vi "Write Microscope Configuration.vi"(8 "error in (no error)":errorcluster, 10 "Microscope Configuration":T1={"Serial Port"="COM2"}, 11 "TE2000 in":refnum<class "TE2000.lvclass">) -> (0 "error out":errorcluster, 3 "TE2000 out":refnum<class "TE2000.lvclass">)   [LabVIEW 2014, in "TE2000.lvlib" / "TE2000.lvclass"]
uses:
  TE2000.lvclass
  Resources/Type Defs/Microscope Configuration.ctl
  TE2000.lvclass/TE2000.ctl
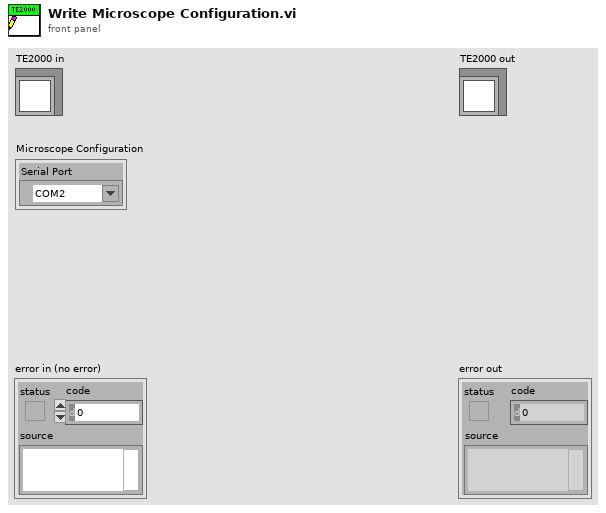
[diagram p1: front panel]
types:
  T1 = typedef "Microscope Configuration.ctl" = cluster{"Serial Port":refnum<visa-resource-name>}
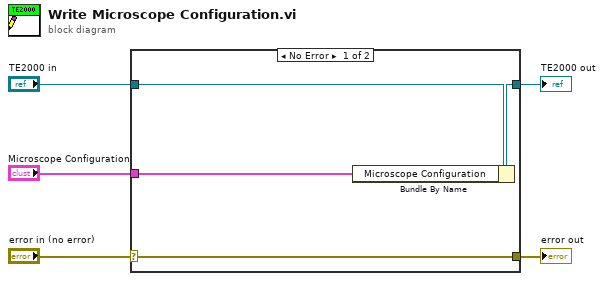
[diagram p0: block diagram]
diagram:
  n1 = case shown="No Error" "error in (no error)" {
    selector: "error in (no error)" -> [w9 w10]
    tunnel: [w9 w10] -> w4
    tunnel: [w7 w11] -> w2
    tunnel: "TE2000 in" -> [w8 w11]
    tunnel: "Microscope Configuration" -> [w6 _]
    frame No Error {
      n2 = Bundle By Name(cluster=w8, "Microscope Configuration"=w6) -> (w7:refnum<class "TE2000.lvclass">)
    }
    frame Error {
    }
  }
  "error out" <- w4
  "TE2000 out" <- w2
